vi "Actor Last Ack.vi"(9 "Nest Error":errorcluster, 10 "Nest Actor":refnum<class "Actor.lvclass">, 11 "Actor Last Ack in":refnum<class "Actor Last Ack.lvclass">) -> (0 "error out":errorcluster, 3 "Actor Last Ack out":refnum<class "Actor Last Ack.lvclass">)   [LabVIEW 2021, in "Actor Last Ack.lvlib" / "Actor Last Ack.lvclass"]
uses:
  Actor Last Ack.lvclass
  LVCAM/Actor/Actor.lvclass
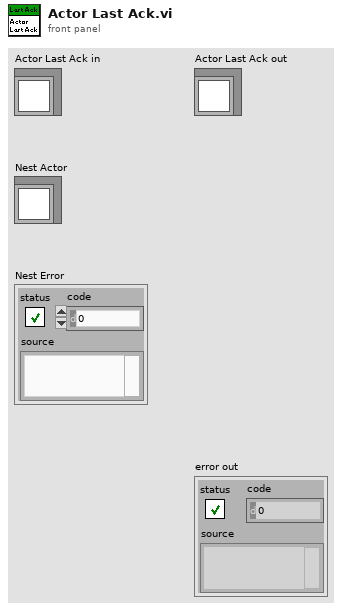
[diagram p1: front panel]
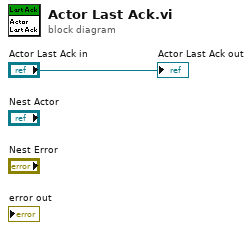
[diagram p0: block diagram]
diagram:
  "Actor Last Ack out" <- "Actor Last Ack in"
